vi "Test_Min_of_3.vi"() -> ()   [LabVIEW 2022 SP3]
panel:
  in  "stop":bool
  in  "input 1":dbl
  in  "input 3":dbl
  in  "input 2":dbl
  out "Numeric out":dbl
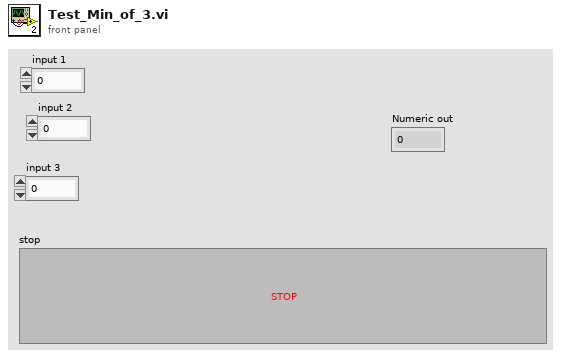
[diagram p1: front panel]
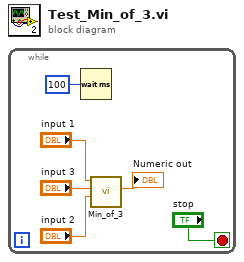
[diagram p0: block diagram]
diagram:
  n1 = while {
    stop <- "stop" stop-if-true
    n2 = Wait (ms)(milliseconds to wait=u32 100) -> ()  [unwired: 1 out]
    n3 = call "Min_of_3.vi"("input 02"="input 2", "input 01"="input 3", "input 03"="input 1") -> ("min"=→"Numeric out":dbl)  [unwired: 7 in, 1 out]
  }
